vi "Sequence.CreateTask.vi"(8 "error in (no error)":errorcluster, 10 "Task Refs":refnum<k24>[](array[refnum]), 11 "Task Ref":refnum<k24>) -> (0 "error out":errorcluster, 3 "Task Ref out":refnum<k24>)   [LabVIEW 2013, in "Simple Sequence Editor.lvlib"]
uses:
  Simple Sequence Editor.lvlib
  NationalInstruments.VeriStand.RealTimeSequenceDefinitionApi
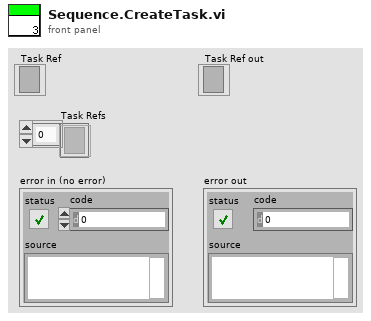
[diagram p1: front panel]
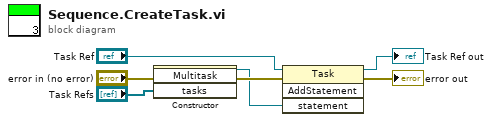
[diagram p0: block diagram]
diagram:
  n1 = constructor class="Multitask"(error in="error in (no error)", "tasks"="Task Refs") -> (reference out=w2:refnum<k24>, error out=w3:errorcluster)  [unwired: 2 in, 2 out]
  n2 = invoke class="Task" method="AddStatement"(reference="Task Ref", error in=w3, "statement"=w2) -> (reference out=→"Task Ref out":refnum<k24>, error out=→"error out":errorcluster)  [unwired: 1 in, 2 out]
